vi "Write Single Coil.vi"(8 "error in (no error)":errorcluster, 9 "value":bool, 10 "address":u16, 11 "MODBUS in":refnum<class "Modbus.lvclass">) -> (0 "error out":errorcluster, 3 "MODBUS Out":refnum<class "Modbus.lvclass">)   [LabVIEW 2020, in "Library Instrument & Equipement.lvlib" / "Library Relay_Board.lvlib" / "Modbus.lvclass"]
doc: "Writes single coil <B>value</B> at specified <B>address</B> (Modbus function code: <B>5</B>)."
uses:
  Modbus.lvclass
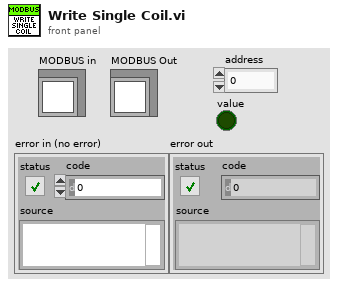
[diagram p1: front panel]
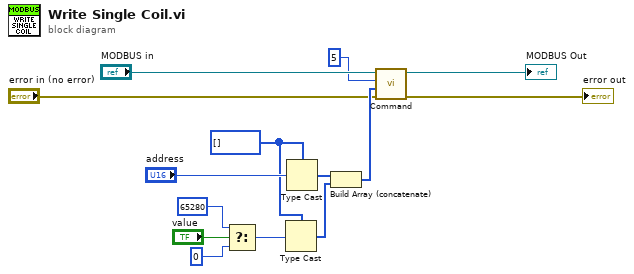
[diagram p0: block diagram]
diagram:
  w4 = u8[] []
  n1 = Select(t=u16 65280 ("unsigned 16bit integer"), s="value", f=u16 0 ("unsigned 16bit integer")) -> (s? t:f=w5:u16)
  n2 = Type Cast(type=w4, x=w5) -> (*(type *) &x=w3:u8[])
  n3 = Type Cast(type=w4, x="address") -> (*(type *) &x=w12:u8[])
  n4 = Build Array (concatenate)(w12, w3) -> (w11:u8[])
  n5 = call-dynamic "Command.vi"("error in (no error)"="error in (no error)", "data in"=w11, "function code"=u8 5 ("function"), "MODBUS in"="MODBUS in") -> ("error out"=→"error out":errorcluster, "MODBUS Out"=→"MODBUS Out":refnum<class "Modbus.lvclass">)  [unwired: 5 in, 1 out]
